vi "测试类型2can应答.vi"(7 "输出切换ID":u8, 8 "输入切换ID":u8) -> (3 "成功？":bool)   [LabVIEW 2010]
uses:
  全局量/全局_配置.vi
panel:
  out "开始时间":dbl format="%#.0f"
  in  "匹配CANID":u32 format="%x"
  out "接收数据":u8[](array[numeric])
  out "超时?":bool
  in  "Baudrate":u32(ring)=1000 caption="K" items=["10"=10, "20"=20, "50"=50, "100"=100, "125"=125, "250"=250, "500"=500, "800"=800, "250"=1000]
  in  "CANPort":u16
  in  "ReadTimeOut":u32=3000 caption="ms"
  in  "Synchronization":i32(ring)=1 items=["Synchronization"=1, "Asynchronization"=0]
  out "Error out":errorcluster {"code" format="%.0x"}
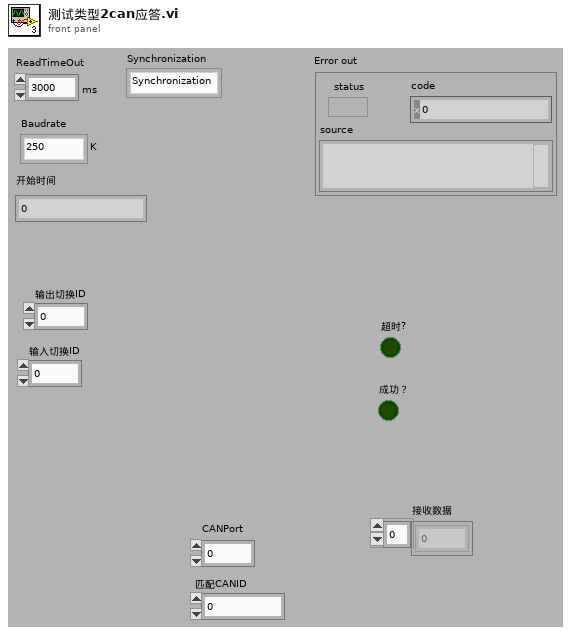
[diagram p1: front panel]
types:
  T1 = cluster{"Internal":u32, "InternalHigh":u32, "Offset":u32, "OffsetHigh":u32, "hEvent":u32}
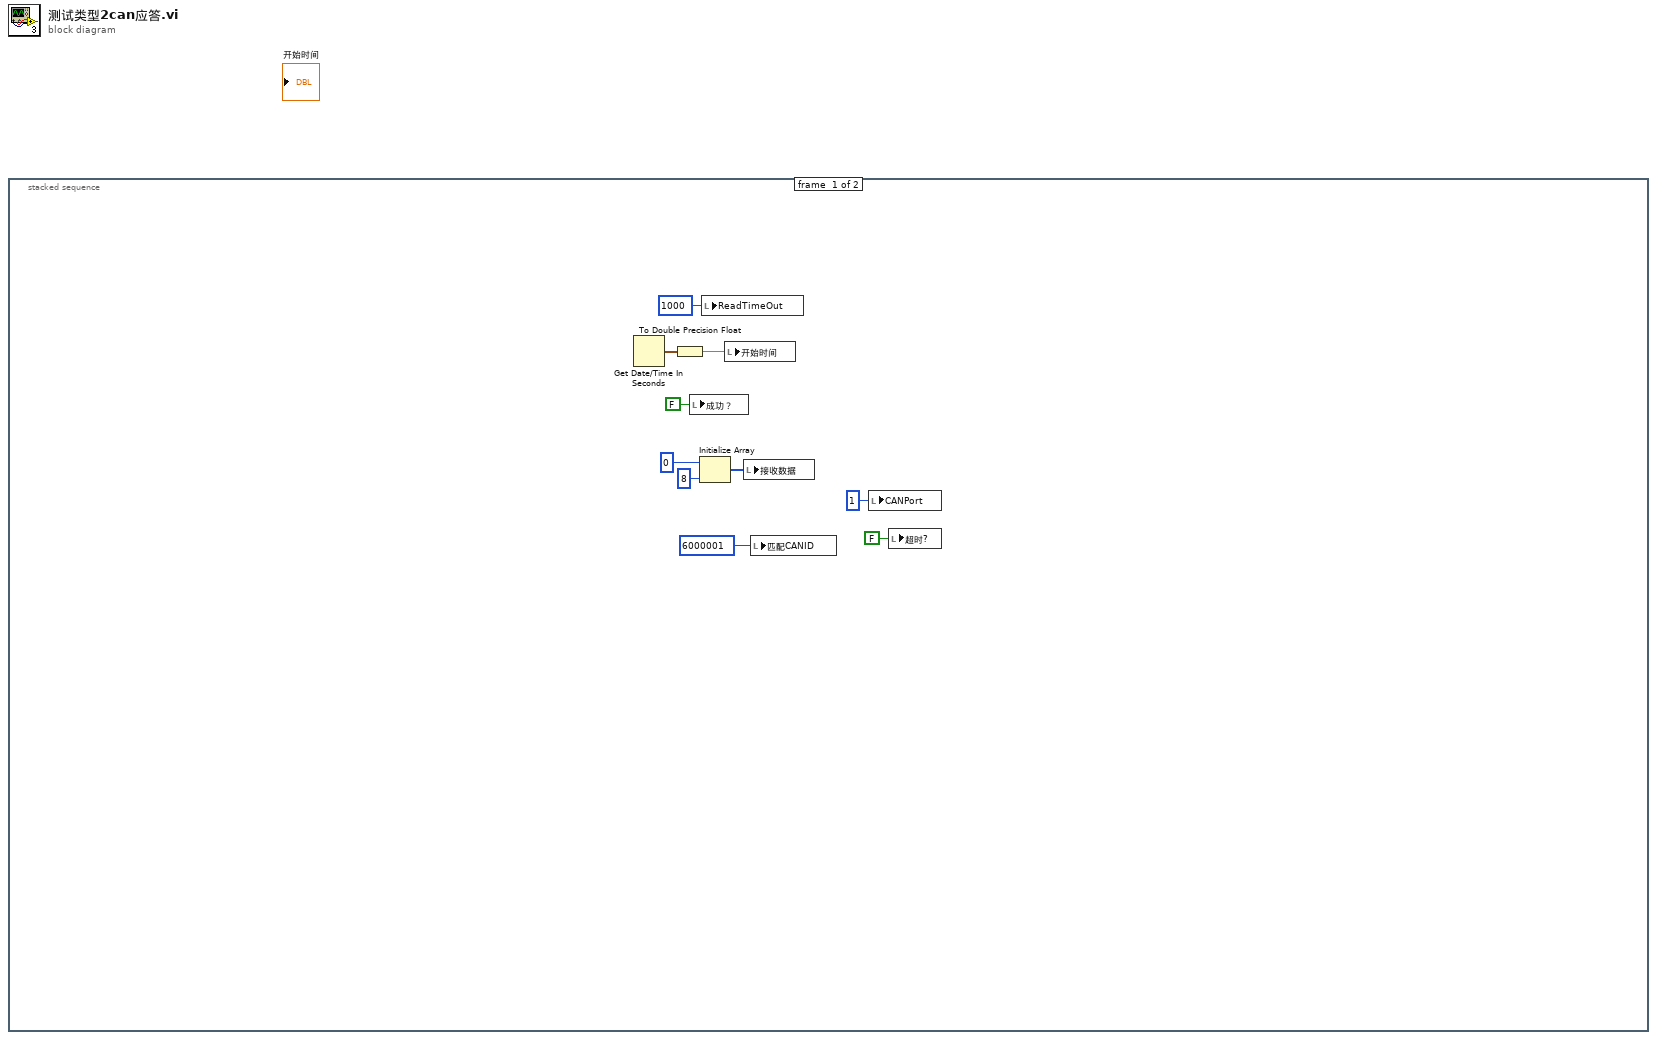
[diagram p0: block diagram]
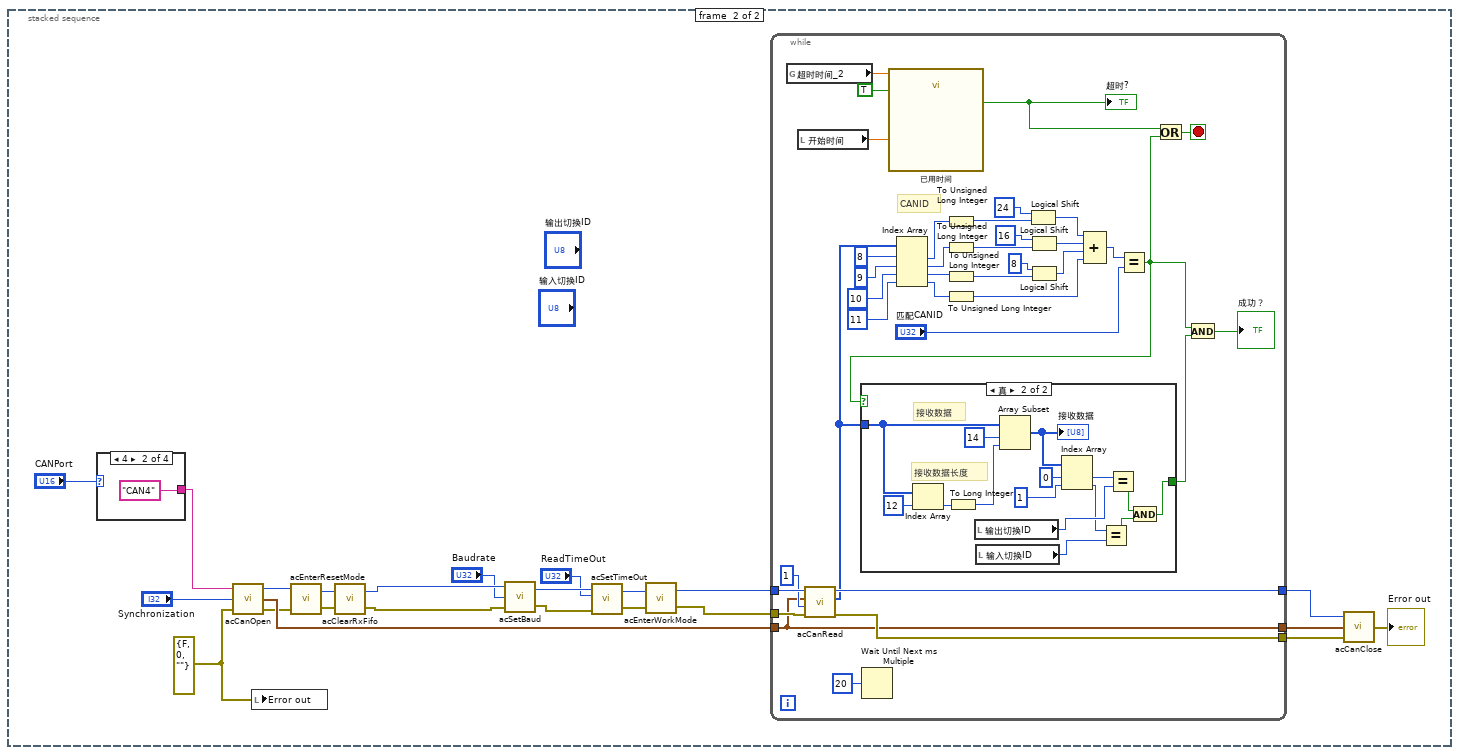
[diagram p2: hidden frame]
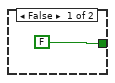
[diagram p3: hidden frame]
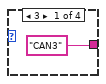
[diagram p4: hidden frame]
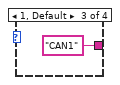
[diagram p5: hidden frame]
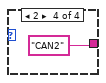
[diagram p6: hidden frame]
diagram:
  n1 = stacked-sequence {
    frame #0 {
      n2 = Get Date/Time In Seconds() -> (seconds since 1Jan1904=w6:timestamp)
      n3 = To Double Precision Float(number=w6) -> (double precision float=w7:dbl)
      n4 = local write "成功？"(FALSE ("成功？")) -> ()
      n5 = Initialize Array(u8 0, 8 ("维数大小")) -> (w5:u8[])
      n6 = local write "ReadTimeOut"(u32 1000 ("ReadTimeOut")) -> ()
      n7 = local write "开始时间"(w7) -> ()
      n8 = local write "接收数据"(w5) -> ()
      n9 = local write "匹配CANID"(6000001 ("维数大小")) -> ()
      n10 = local write "CANPort"(u16 1 ("CANPort")) -> ()
      n11 = local write "超时?"(FALSE ("超时?")) -> ()
    }
    frame #1 {
      w27 = errorcluster {"status"=FALSE, "code"=0, "source"=""} ("Error in")
      n12 = case shown="4" "CANPort" {
        tunnel: ["CAN3" "CAN4" "CAN1" "CAN2"] -> w12
        frame 3 {
        }
        frame 4 {
        }
        frame 1, Default {
        }
        frame 2 {
        }
      }
      n13 = call "acCanOpen.vi"("Error in"=w27, "Synchronization"="Synchronization", "CANPort"=w12) -> ("Error out"=w28:errorcluster, "Overlapped"=w31:T1, "Handle"=w29:u32)
      n14 = local write "Error out"(w27) -> ()
      n15 = call "acEnterResetMode.vi"("Error in"=w28, "Handle  in"=w29) -> ("Error out"=w22:errorcluster, "Handle out"=w21:u32)
      n16 = call "acClearRxFifo.vi"("Error in"=w22, "Handle  in"=w21) -> ("Error out"=w19:errorcluster, "Handle out"=w20:u32)
      n17 = call "acSetBaud.vi"("Error in"=w19, "Baudrate"="Baudrate", "Handle  in"=w20) -> ("Error out"=w24:errorcluster, "Handle out"=w25:u32)
      n18 = call "acSetTimeOut.vi"("Error in"=w24, "Read TimeOut"="ReadTimeOut", "Handle  in"=w25) -> ("Error out"=w17:errorcluster, "Handle out"=w18:u32)  [unwired: 1 in]
      n19 = call "acEnterWorkMode.vi"("Error in"=w17, "Handle  in"=w18) -> ("Error out"=w15:errorcluster, "Handle out"=w16:u32)
      n20 = while {
        tunnel: [w69] -> w32
        tunnel: w31 -> [w64]
        tunnel: [w68] -> w30
        tunnel: w16 -> [w67]
        tunnel: w15 -> [w66]
        tunnel: [w64] -> w11
        stop <- w60 stop-if-true
        # "CANID"
        n21 = global read "全局_配置.vi" "超时时间_2"() -> (w62:dbl)
        n22 = local read "开始时间"() -> (w61:dbl)
        n23 = call "acCanRead.vi"("Error in"=w66, "ReadCount"=u32 1 ("接收CAN帧数 2"), "Overlapped"=w64, "Handle  in"=w67) -> ("Error out"=w68:errorcluster, "MSG"=w38:u8[], "Handle out"=w69:u32)  [unwired: 1 out]
        n24 = Wait Until Next ms Multiple(millisecond multiple=u32 20 ("毫秒倍数")) -> ()  [unwired: 1 out]
        n25 = call "已用时间"("Time Target (s)"=w62, "Reset"=TRUE, "Set Start Time (s)"=w61) -> ("Time has Elapsed"=w34:bool)  [unwired: 9 in, 7 out]
        "超时?" <- w34
        n26 = Index Array(array=w38, index #1=8 ("索引"), index #2=9 ("索引"), index #3=10 ("索引"), index #4=11 ("索引")) -> (element #1=w45:u8, element #2=w44:u8, element #3=w41:u8, element #4=w40:u8)
        n27 = To Unsigned Long Integer(number=w45) -> (unsigned 32bit integer=w46:u32)
        n28 = To Unsigned Long Integer(number=w44) -> (unsigned 32bit integer=w43:u32)
        n29 = To Unsigned Long Integer(number=w41) -> (unsigned 32bit integer=w42:u32)
        n30 = To Unsigned Long Integer(number=w40) -> (unsigned 32bit integer=w39:u32)
        n31 = Logical Shift(y=i8 24, x=w46) -> (x << y=w50:u32)
        n32 = Logical Shift(y=i8 16, x=w43) -> (x << y=w51:u32)
        n33 = Logical Shift(y=i8 8, x=w42) -> (x << y=w49:u32)
        n34 = Compound Arithmetic op=ADD(w50, w51, w49, w39) -> (w48:u32)
        n35 = Equal?(x=w48, y="匹配CANID") -> (x = y?=w37:bool)
        n36 = case shown="真" w37 {
          tunnel: w38 -> [_ w81]
          tunnel: [FALSE w71] -> w36
          frame False {
          }
          frame True {
            # "接收数据"
            # "接收数据长度"
            n37 = Index Array(array=w81, index=12 ("索引")) -> (element=w83:u8)
            n38 = To Long Integer(number=w83) -> (32bit integer=w82:i32)
            n39 = local read "输出切换ID"() -> (w76:u8)
            n40 = local read "输入切换ID"() -> (w74:u8)
            n41 = Array Subset(array=w81, index=14 ("索引"), length=w82) -> (w80:u8[])
            "接收数据" <- w80
            n42 = Index Array(array=w80, index #1=0 ("索引"), index #2=1 ("索引")) -> (element #1=w78:u8, element #2=w75:u8)
            n43 = Equal?(x=w75, y=w74) -> (x = y?=w72:bool)
            n44 = Equal?(x=w78, y=w76) -> (x = y?=w73:bool)
            n45 = And(x=w73, y=w72) -> (x .and. y?=w71:bool)
          }
        }
        n46 = Or(x=w34, y=w37) -> (x .or. y?=w60:bool)
        n47 = And(x=w37, y=w36) -> (x .and. y?=→"成功？":bool)
      }
      n48 = call "acCanClose.vi"("Error in"=w30, "Overlapped"=w11, "Handle  in"=w32) -> ("Error out"=→"Error out":errorcluster)
    }
  }
